vi "ReadWriteCounterFile.vi"(10 "Counter File Options":T1) -> (0 "error out":errorcluster, 2 "Measurements Done":i64)   [LabVIEW 2021]
uses:
  Enums/Counter_File_Options.ctl
  <vilib>/Utility/file.llb/Read Delimited Spreadsheet (I64).vi
  <vilib>/Utility/file.llb/Write Delimited Spreadsheet (I64).vi
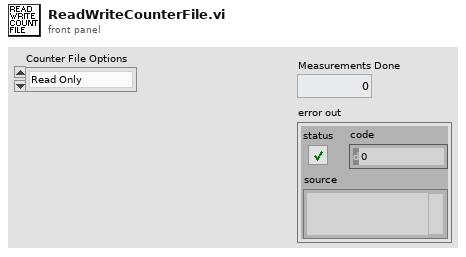
[diagram p1: front panel]
types:
  T1 = typedef "Counter_File_Options.ctl" = enum16{"Read Only", "Increment", "Reset"}
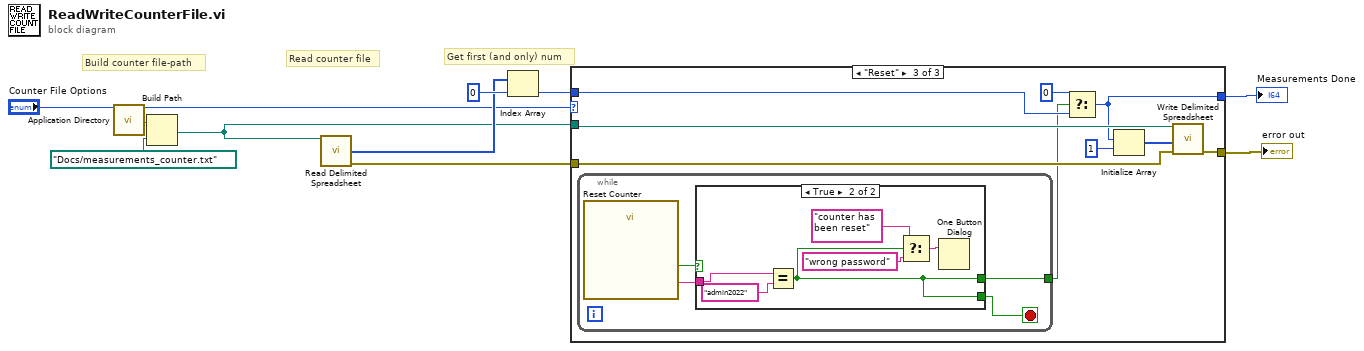
[diagram p0: block diagram]
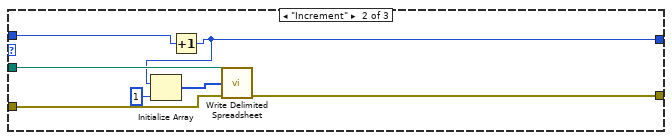
[diagram p3: hidden frame]
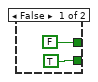
[diagram p4: hidden frame]
diagram:
  # "Build counter file-path"
  # "Get first (and only) num"
  # "Read counter file"
  n1 = call <vilib>:"Application Directory.vi"() -> ("Application Directory"=w9:path)
  n2 = Build Path(base path=w9, name or relative path=path "Docs/measurements_counter.txt") -> (appended path=w2:path)
  n3 = call-poly <vilib>:"Read Delimited Spreadsheet.vi"("file path (dialog if empty)"=w2) -> ("first row"=w8:i64[], "error out"=w6:errorcluster)  [unwired: 9 in, 4 out]
  n4 = Index Array(array=w8, index=0) -> (element=w4:i64)
  n5 = case shown="\"Reset\"" "Counter File Options" {
    tunnel: w2 -> [_ w19 w25]
    tunnel: w6 -> [w11 w18 w28]
    tunnel: [w11 w17 w27] -> w5
    tunnel: w4 -> [w12 w16 w23]
    tunnel: [w12 w15 w20] -> w3
    frame "Read Only", Default {
    }
    frame "Increment" {
      n6 = Increment(x=w16) -> (x+1=w15:i64)
      n7 = Initialize Array(w15, 1 ("dimension size")) -> (w14:i64[])
      n8 = call-poly <vilib>:"Write Delimited Spreadsheet.vi"("file path (dialog if empty)"=w19, "1D data"=w14, "error in (no error)"=w18) -> ("error out"=w17:errorcluster)  [unwired: 11 in, 1 out]
    }
    frame "Reset" {
      n9 = while {
        tunnel: [w30] -> w22
        stop <- w29 stop-if-true
        n10 = call "Reset Counter"() -> ("Password"=w31:string, "Reset"=w32:bool)  [unwired: 17 in, 1 out]
        n11 = case shown="True" w32 {
          tunnel: w31 -> [_ w39]
          tunnel: [FALSE w35] -> w30
          tunnel: [TRUE w35] -> w29
          frame False {
          }
          frame True {
            n12 = Equal?(x=w39, y="admin2022") -> (x = y?=w35:bool)
            n13 = Select(t="counter has been reset" ("message"), s=w35, f="wrong password" ("message")) -> (s? t:f=w36:string)
            n14 = One Button Dialog(message=w36) -> ()  [unwired: 1 in, 1 out]
          }
        }
      }
      n15 = Select(t=i64 0, s=w22, f=w23) -> (s? t:f=w20:i64)
      n16 = Initialize Array(w20, 1 ("dimension size")) -> (w24:i64[])
      n17 = call-poly <vilib>:"Write Delimited Spreadsheet.vi"("file path (dialog if empty)"=w25, "1D data"=w24, "error in (no error)"=w28) -> ("error out"=w27:errorcluster)  [unwired: 11 in, 1 out]
    }
  }
  "Measurements Done" <- w3
  "error out" <- w5
